vi "Verify Data Types.vi"(1 "text":string) -> (0 "Picture":picture)   [LabVIEW 2010]
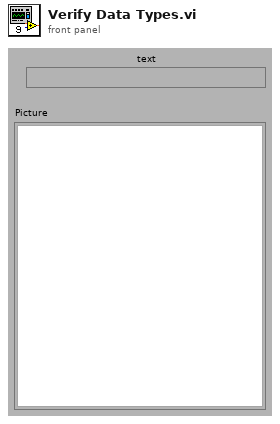
[diagram p1: front panel]
types:
  T1 = cluster{"left":i16, "top":i16, "right":i16, "bottom":i16}
  T2 = cluster{"horizontal":enum16{"left", "center", "right"}, "vertical":enum16{"top", "center", "bottom"}}
  T3 = enum16{"User-specified Font", "Application Font", "System Font", "Dialog Font"}
  T4 = cluster{"Font Name:":string, "Size":i16, "Strikeout?":bool, "Italic?":bool, "Underline?":bool, "Outline?":bool, "Shadow?":bool, "Bold?":bool}
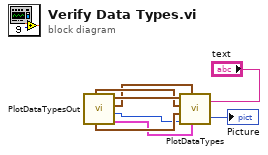
[diagram p0: block diagram]
diagram:
  n1 = call "PlotDataTypesOut.vi"() -> ("point 2"=w7:cluster{"x":i16, "y":i16}, "rect"=w6:T1, "point"=w8:cluster{"x":i16, "y":i16}, "alignment"=w5:T2, "desired font"=w3:T3, "user-specified font"=w4:T4)  [unwired: 3 out]
  n2 = call "PlotDataTypes.vi"("text"="text", "user-specified font"=w4, "alignment"=w5, "desired font"=w3, "rect"=w6, "point 2"=w7, "point"=w8) -> ("Picture"=→"Picture":picture)
